vi "Bin_Cyclic_Signal.vi"(5 "Max Time":dbl, 6 "LDA Data? (False)":bool, 7 "Transit Time":dbl[](array[numeric]), 8 "dt":dbl, 9 "No of bins":i32, 10 "Time":dbl[](array[numeric]), 11 "Eng Values":dbl[](array[numeric])) -> (2 "SJ Results":T1)   [LabVIEW 2011]
uses:
  <vilib>/Analysis/NI_AALBase.lvlib
  <vilib>/Analysis/1siggen.llb/Ramp Pattern by Samples.vi
  <vilib>/Analysis/NI_AALPro.lvlib
  <vilib>/Analysis/5stat.llb/RMS (DBL).vi
  Controls/SJ_Results_Cluster.ctl
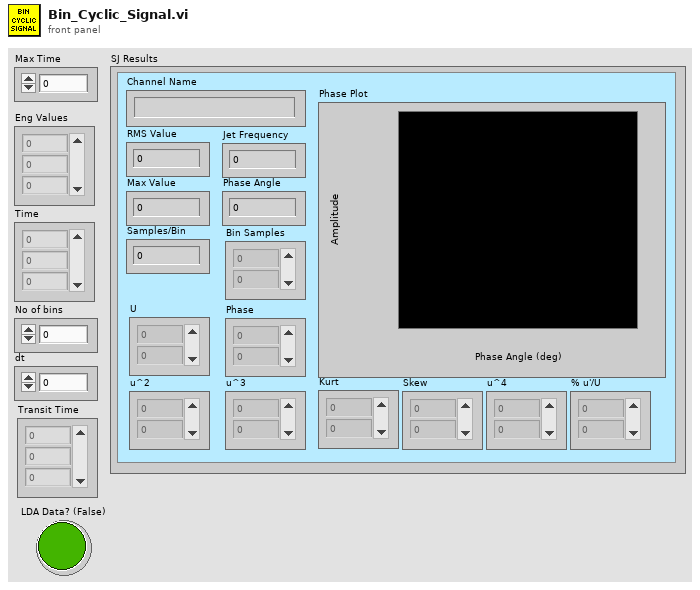
[diagram p1: front panel]
types:
  T1 = typedef "SJ_Results_Cluster.ctl" = cluster{"U":dbl[], "u^2":dbl[], "u^3":dbl[], "u^4":dbl[], "Skew":dbl[], "Kurt":dbl[], "% u'/U":dbl[], "Phase":dbl[], "Bin Samples":dbl[], "Phase Plot":cluster{"Phase Angle":dbl[], dbl[]}, "Channel Name":string, "Max Value":dbl, "RMS Value":dbl, "Phase Angle":dbl, "Jet Frequency":dbl, "Samples/Bin":i32}
  T2 = cluster{"Ramp Pattern":dbl[], "Phase Averaged Signal":dbl[]}
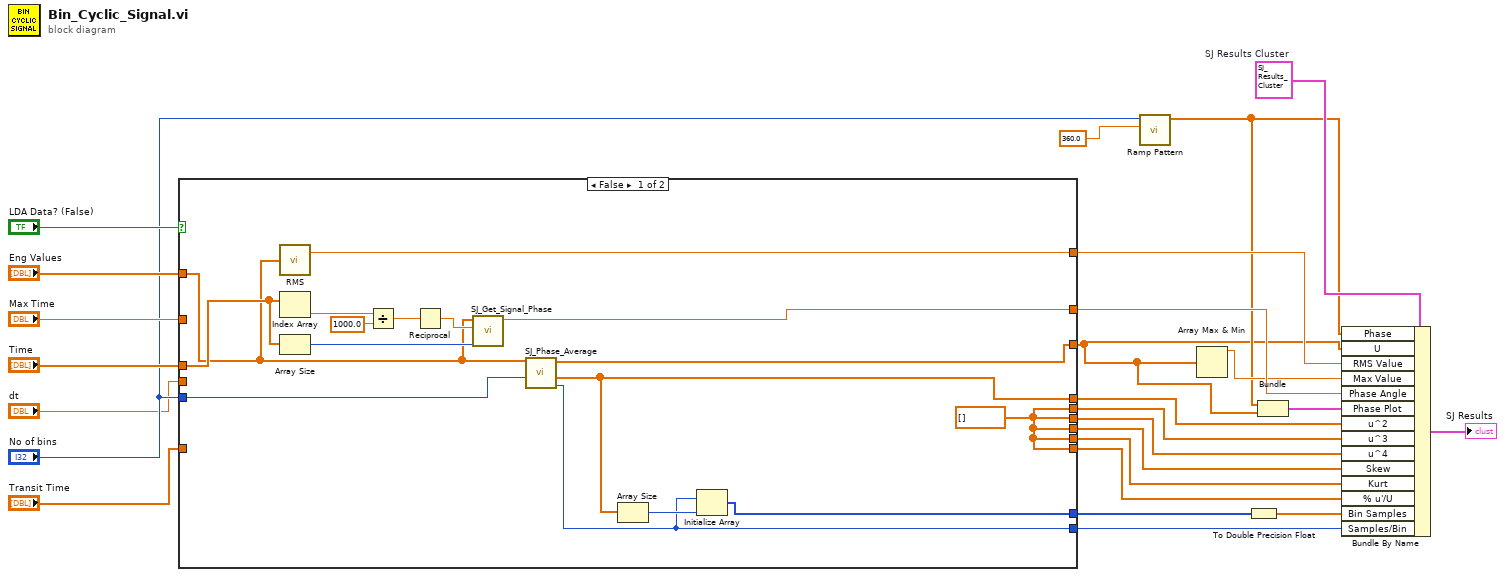
[diagram p0: block diagram]
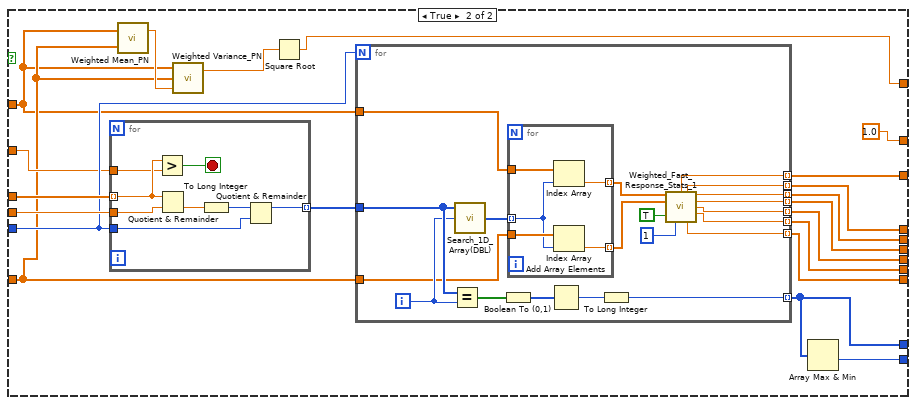
[diagram p2: hidden frame]
diagram:
  w18 = T1 {"U"=[], "u^2"=[], "u^3"=[], "u^4"=[], "Skew"=[], "Kurt"=[], "% u'/U"=[], "Phase"=[], "Bin Samples"=[], "Phase Plot"={"Phase Angle"=[], []}, "Channel Name"="", "Max Value"=0.0, "RMS Value"=0.0, "Phase Angle"=0.0, "Jet Frequency"=0.0, "Samples/Bin"=0}  # SJ Results Cluster
  n1 = case shown="False" "LDA Data? (False)" {
    tunnel: "No of bins" -> [w41 w59]
    tunnel: "Eng Values" -> [w26 w44]
    tunnel: "Time" -> [w27 w61]
    tunnel: "dt" -> [_ w60]
    tunnel: "Max Time" -> [_ w58]
    tunnel: "Transit Time" -> [_ w45]
    tunnel: [w33 w55] -> w4
    tunnel: [w35 1.0 ("Phase Angle")] -> w17
    tunnel: [w34 w42] -> w16
    tunnel: [w31 w54] -> w10
    tunnel: [w32 w53] -> w9
    tunnel: [w32 w52] -> w8
    tunnel: [w32 w51] -> w7
    tunnel: [w32 w50] -> w6
    tunnel: [w32 w49] -> w5
    tunnel: [w28 w48] -> w3
    tunnel: [w29 w47] -> w2
    frame False {
      w32 = dbl[] []
      n2 = call-poly <vilib>:"RMS.vi"("X"=w26) -> ("rms value"=w34:dbl)  [unwired: 1 out]
      n3 = Index Array(array=w27) -> (element=w40:dbl)  [unwired: 1 in]
      n4 = Array Size(array=w27) -> (size(s)=w36:i32)
      n5 = Divide(x=w40, y=1000.0) -> (x/y=w38:dbl)
      n6 = Reciprocal(x=w38) -> (1/x=w37:dbl)
      n7 = call "SJ_Get_Signal_Phase.vi"("No of Analogue Samples"=w36, "Actual Sampling Frequency"=w37, "Signal"=w26) -> ("Phase Angle"=w35:dbl)  [unwired: 8 in]
      n8 = call "SJ_Phase_Average.vi"("No. of Bins"=w41, "1D Signal"=w26) -> ("Samples per Bin"=w29:i32, "Variance"=w31:dbl[], "Phase Averaged Signal"=w33:dbl[])  [unwired: 6 in, 1 out]
      n9 = Array Size(array=w31) -> (size(s)=w30:i32)
      n10 = Initialize Array(w29, w30) -> (w28:i32[])
    }
    frame True {
      n11 = for {
        tunnel: w61 -> [w89] mode=indexing
        tunnel: w60 -> [w94]
        tunnel: w59 -> [w90]
        tunnel: [w91] -> w57 mode=indexing
        tunnel: w58 -> [w88]
        stop <- w87 stop-if-true
        n12 = Greater?(x=w89, y=w88) -> (0:w87:bool)
        n13 = Quotient & Remainder(x=w89, y=w94) -> (floor(x/y)=w93:dbl)  [unwired: 1 out]
        n14 = To Long Integer(number=w93) -> (32bit integer=w92:i32)
        n15 = Quotient & Remainder(x=w92, y=w90) -> (x-y*floor(x/y)=w91:i32)  [unwired: 1 out]
      }
      n16 = call "Weighted Mean_PN.vi"("weights"=w45, "1D data"=w44) -> ("Weighted mean"=w46:dbl)  [unwired: 1 in]
      n17 = call "Weighted Variance_PN.vi"("Weighted mean"=w46, "weights"=w45, "1D data"=w44) -> ("Weighted variance"=w43:dbl)  [unwired: 1 in]
      n18 = Square Root(x=w43) -> (sqrt(x)=w42:dbl)
      n19 = for {
        N: w59 -> [_]
        tunnel: w57 -> [w78]
        tunnel: w44 -> [w76]
        tunnel: w45 -> [w74]
        tunnel: [w69] -> w55 mode=indexing
        tunnel: [w68] -> w54 mode=indexing
        tunnel: [w67] -> w53 mode=indexing
        tunnel: [w66] -> w52 mode=indexing
        tunnel: [w65] -> w51 mode=indexing
        tunnel: [w64] -> w50 mode=indexing
        tunnel: [w63] -> w49 mode=indexing
        tunnel: [w62] -> w48 mode=indexing
        i -> [w77]
        n20 = Equal?(x=w78, y=w77) -> (x = y?=w81:bool[])
        n21 = call "Search_1D_Array(DBL).vi"("Array"=w78, "Element Data"=w77) -> ("Indicies of Elements"=w75:i32[])  [unwired: 7 in]
        n22 = Boolean To (0,1)(Boolean=w81) -> (0, 1=w80:i16[])
        n23 = for {
          tunnel: w76 -> [w86]
          tunnel: w75 -> [w82] mode=indexing
          tunnel: w74 -> [w85]
          tunnel: [w84] -> w71 mode=indexing
          tunnel: [w83] -> w70 mode=indexing
          n24 = Index Array(array=w86, index=w82) -> (element=w83:dbl)
          n25 = Index Array(array=w85, index=w82) -> (element=w84:dbl)
        }
        n26 = Add Array Elements(numeric array=w80) -> (sum=w79:i16)
        n27 = To Long Integer(number=w79) -> (32bit integer=w62:i32)
        n28 = call "Weighted_Fast_Response_Stats_1.vi"("U"=w70, "Weighting"=w71, "Use Weighting?"=TRUE, "Block No"=1) -> ("U"=w69:dbl, "u^2"=w68:dbl, "u^3"=w67:dbl, "u^4"=w66:dbl, "Skew"=w65:dbl, "Kurt"=w64:dbl, "% u'/U"=w63:dbl)  [unwired: 4 in, 1 out]
      }
      n29 = Array Max & Min(array=w48) -> (min value=w47:i32)  [unwired: 3 out]
    }
  }
  n30 = call-poly <vilib>:"Ramp Pattern.vi"("end"=360.0, "samples"="No of bins") -> ("Ramp Pattern"=w14:dbl[])  [unwired: 8 in, 1 out]
  n31 = Array Max & Min(array=w4) -> (max value=w15:dbl)  [unwired: 3 out]
  n32 = To Double Precision Float(number=w3) -> (double precision float=w1:dbl[])
  n33 = Bundle("Ramp Pattern"=w14, "Phase Averaged Signal"=w4) -> (w13:T2)  [unwired: 1 in]
  n34 = Bundle By Name(cluster=w18, "Phase"=w14, "U"=w4, "RMS Value"=w16, "Max Value"=w15, "Phase Angle"=w17, "Phase Plot"=w13, "u^2"=w10, "u^3"=w9, "u^4"=w8, "Skew"=w7, "Kurt"=w6, "% u'/U"=w5, "Bin Samples"=w1, "Samples/Bin"=w2) -> (→"SJ Results":T1)
